vi "svx_Generate Shock Pulse.vi"(8 "error in (no error)":errorcluster, 11 "simulated shock":T1={"signal type"=enum."Half-sine pulse", "pulse duration"=0.05, "amplitude"=1.0, "sampling info"={"sampling frequency"=51200.0, "# of samples"=5120.0}} {"sampling info"."# of samples" min=100.0; "sampling info"."sampling frequency" min=0.0 format="%.2p"; "amplitude" min=0.0 format="%.2f"; "pulse duration" min=0.0 format="%.1p"}) -> (0 "error out":errorcluster, 2 "time record [ms]":dbl=100.0 format="%.2f", 3 "Waveform Graph":waveform(dbl)(graph), 5 "pulse duration [ms]":dbl=100.0 format="%.2f")   [LabVIEW 2017]
doc: "Simulates a shock pulse."
uses:
  <vilib>/Waveform/WDTOps.llb/WDT Get Final Time Value DBL.vi
  <vilib>/Waveform/WDTOps.llb/WDT Append Waveforms DBL.vi
  <vilib>/measure/NI_MABase.lvlib
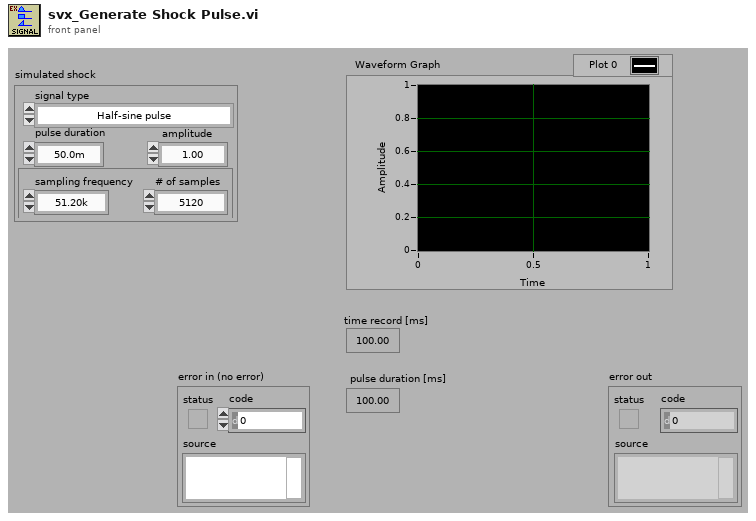
[diagram p1: front panel]
types:
  T1 = cluster{"signal type":enum16{"Half-sine pulse", "Rectangular pulse", "Sawtooth pulse"}, "pulse duration":dbl, "amplitude":dbl, "sampling info":cluster{"sampling frequency":dbl, "# of samples":dbl}}
  T2 = enum16{"Half-sine pulse", "Rectangular pulse", "Sawtooth pulse"}
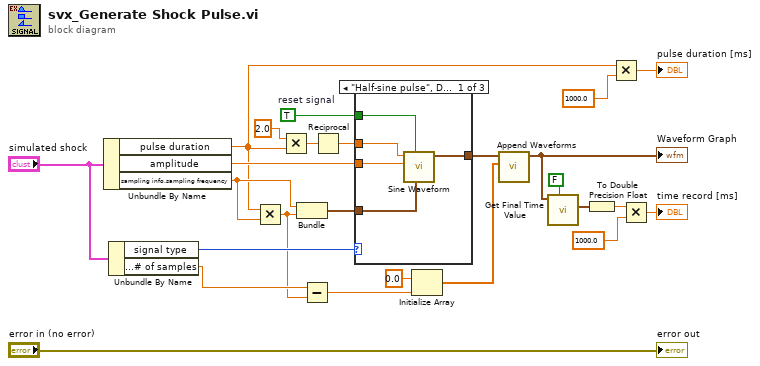
[diagram p0: block diagram]
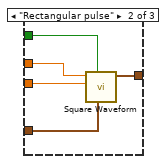
[diagram p2: hidden frame]
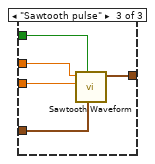
[diagram p3: hidden frame]
diagram:
  w4 = TRUE  # reset signal
  n1 = Unbundle By Name("simulated shock") -> ("pulse duration"=w1:dbl, "amplitude"=w19:dbl, "sampling info.sampling frequency"=w18:dbl)
  n2 = Unbundle By Name("simulated shock") -> ("signal type"=w25:T2, "sampling info.# of samples"=w17:dbl)
  n3 = Multiply(x=w1, y=w18) -> (x*y=w16:dbl)
  n4 = Multiply(x=2.0, y=w1) -> (x*y=w22:dbl)
  n5 = Bundle("sampling frequency"=w18, w16) -> (w20:cluster{"sampling frequency":dbl, dbl})  [unwired: 1 in]
  n6 = Subtract(x=w17, y=w16) -> (x-y=w14:dbl)
  n7 = Reciprocal(x=w22) -> (1/x=w21:dbl)
  n8 = case shown="\"Half-sine pulse\", Default" w25 {
    tunnel: w19 -> [w30 w35 w40]
    tunnel: w21 -> [w29 w33 w39]
    tunnel: w20 -> [w28 w34 w38]
    tunnel: [w27 w32 w37] -> w15
    tunnel: w4 -> [w26 w31 w36]
    frame "Half-sine pulse", Default {
      n9 = call <vilib>:"Sine Waveform.vi"("sampling info"=w28, "reset signal"=w26, "amplitude"=w30, "frequency"=w29) -> ("signal out"=w27:waveform(dbl))  [unwired: 6 in, 1 out]
    }
    frame "Rectangular pulse" {
      n10 = call <vilib>:"Square Waveform.vi"("sampling info"=w34, "reset signal"=w31, "amplitude"=w35, "frequency"=w33) -> ("signal out"=w32:waveform(dbl))  [unwired: 6 in, 1 out]
    }
    frame "Sawtooth pulse" {
      n11 = call <vilib>:"Sawtooth Waveform.vi"("sampling info"=w38, "reset signal"=w36, "amplitude"=w40, "frequency"=w39) -> ("signal out"=w37:waveform(dbl))  [unwired: 6 in, 1 out]
    }
  }
  n12 = Initialize Array(0.0 ("element"), w14) -> (w12:dbl[])
  n13 = call-poly <vilib>:"Append Waveforms.vi"("waveform B"=w12, "waveform A"=w15) -> ("waveform out"=w8:waveform(dbl))  [unwired: 8 in, 1 out]
  "Waveform Graph" <- w8
  n14 = call-poly <vilib>:"Get Final Time Value.vi"("open interval? (T)"=FALSE, "waveform in"=w8) -> ("tf"=w7:timestamp)  [unwired: 7 in, 2 out]
  n15 = To Double Precision Float(number=w7) -> (double precision float=w6:dbl)
  n16 = Multiply(x=w1, y=1000.0) -> (x*y=→"pulse duration [ms]":dbl)
  n17 = Multiply(x=w6, y=1000.0) -> (x*y=→"time record [ms]":dbl)
  "error out" <- "error in (no error)"
